vi "fit-function_v03__with_pars_and_eval_node_wrapper.vi"(9 "coefficients":dbl[](array[numeric])=[12.849354442227447, 5.866421178332907, 12.080788064739096, 5.80910915007397, 1224.8335576996235, 9.529730177350924] format="%.6f", 10 "x":dbl[](array[numeric]), 11 "formula":string="y=a0*exp(-x^2/a1^2)+a2*exp(-(x-a3)^2/a4^2);") -> (2 "function\nvariables":string[](array[string]), 3 "y":dbl[](graph))   [LabVIEW 2010]
panel:
  out "error out":errorcluster
  in  "error in":errorcluster
  # "Needs:\na funtion in C syntax with variables a0, a1, a2, ...\ncoefficients for the variables\nx values\n\nReturns:\ny values\n\n\nif the number of coefficients supplied don't\nmatch the number of variables in the formula,\nthe array of coefficients will be pruned or fulled\nup with  0's."
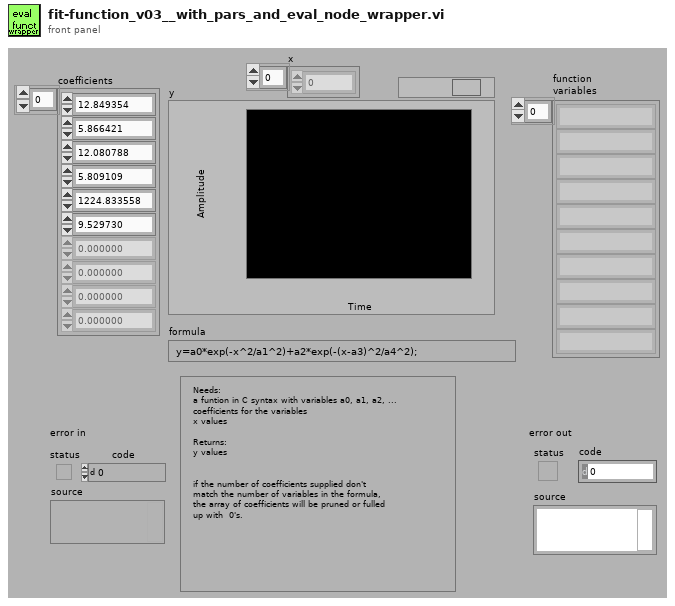
[diagram p1: front panel]
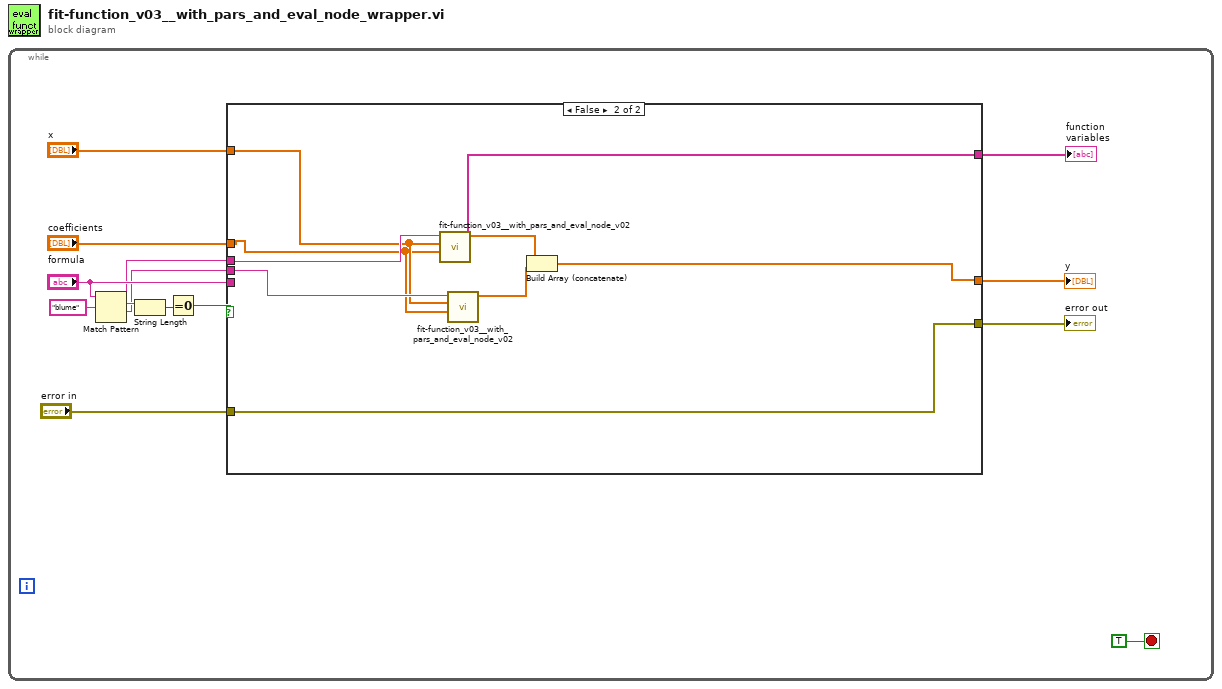
[diagram p0: block diagram]
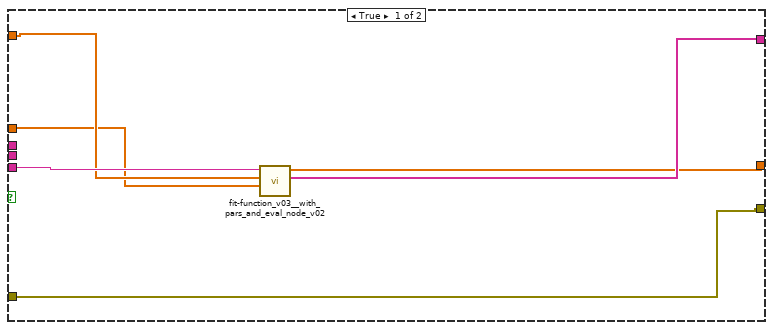
[diagram p2: hidden frame]
diagram:
  n1 = while {
    stop <- TRUE stop-if-true
    n2 = Match Pattern(string="formula", regular expression="blume") -> (before substring=w2:string, match substring=w5:string, after substring=w1:string)  [unwired: 1 in, 1 out]
    n3 = String Length(string=w5) -> (length=w4:i32)
    n4 = Equal To 0?(x=w4) -> (x = 0?=w3:bool)
    n5 = case shown="False" w3 {
      tunnel: [w15 w23] -> w13
      tunnel: "coefficients" -> [w17 w26]
      tunnel: "x" -> [w18 w27]
      tunnel: [w16 w21] -> w10
      tunnel: "error in" -> [w20 w22]
      tunnel: [w20 w22] -> w8
      tunnel: "formula" -> [w19 _]
      tunnel: w2 -> [_ w29]
      tunnel: w1 -> [_ w28]
      frame True {
        n6 = call "fit-function_v03__with_pars_and_eval_node_v02.vi"("coefficients"=w17, "x"=w18, "formula"=w19) -> ("parameter"=w16:string[], "y"=w15:dbl[])  [unwired: 7 in]
      }
      frame False {
        n7 = call "fit-function_v03__with_pars_and_eval_node_v02.vi"("coefficients"=w26, "x"=w27, "formula"=w29) -> ("parameter"=w21:string[], "y"=w25:dbl[])  [unwired: 7 in]
        n8 = call "fit-function_v03__with_pars_and_eval_node_v02.vi"("coefficients"=w26, "x"=w27, "formula"=w28) -> ("y"=w24:dbl[])  [unwired: 7 in, 1 out]
        n9 = Build Array (concatenate)(w25, w24) -> (w23:dbl[])
      }
    }
    "function\nvariables" <- w10
    "y" <- w13
    "error out" <- w8
  }
